vi "LEIN to Encapsulation.vi"(0 "LEIN Variation":T1, 7 "CMD":T2={"SID"=0, "ANF"=FALSE, "CMD"=enum."TASK", "DATA"=[]}, 11 "error in (no error)":errorcluster) -> (2 "Header":u16, 3 "Data":u8[](array[numeric]), 8 "Data and header":u8[](array[numeric]), 14 "Data Length":u32, 15 "error out":errorcluster)   [LabVIEW 2011]
uses:
  Defenitions/LEIN CMD Cluster.ctl
  Defenitions/LEIN CMD List.ctl
  Defenitions/LEIN Structure variations.ctl
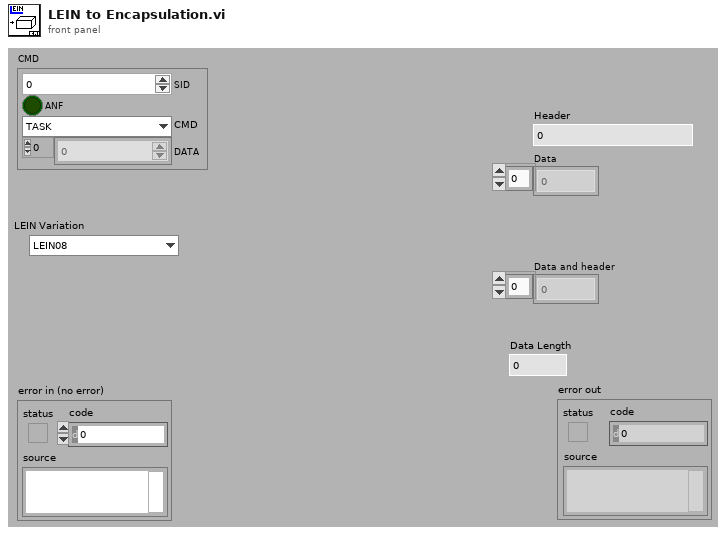
[diagram p1: front panel]
types:
  T1 = typedef "LEIN Structure variations.ctl" = enum16{"LEIN08", "LEIN31", "LEIN63"}
  T2 = typedef "LEIN CMD Cluster.ctl" = cluster{"SID":u8, "ANF":bool, "CMD":T3, "DATA":u8[]}
  T3 = typedef "LEIN CMD List.ctl" = enum8{"ACTI", "TASK", "RES0", "STAT", "RES1", "RES2", "RES3", "USER"}
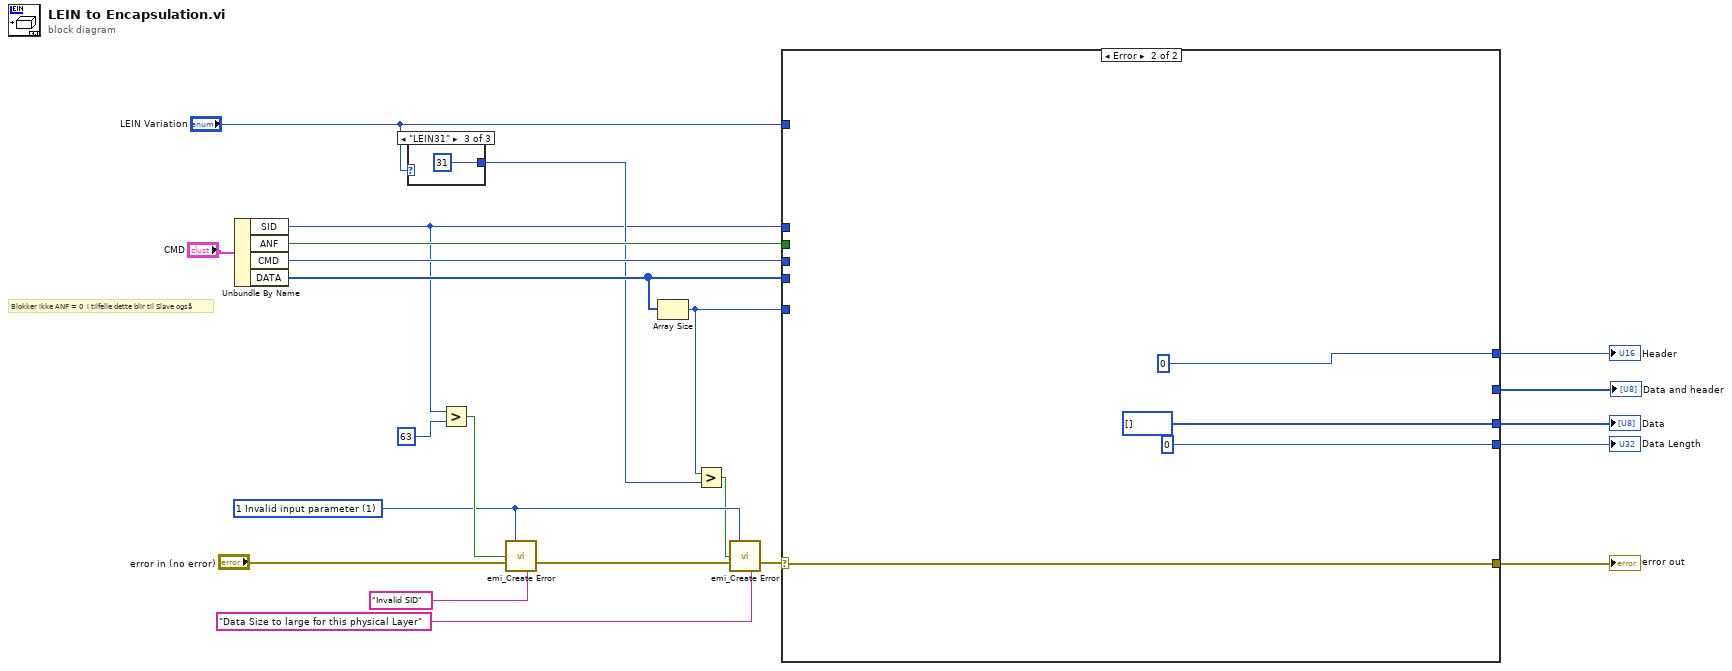
[diagram p0: block diagram]
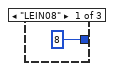
[diagram p2: hidden frame]
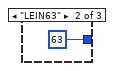
[diagram p3: hidden frame]
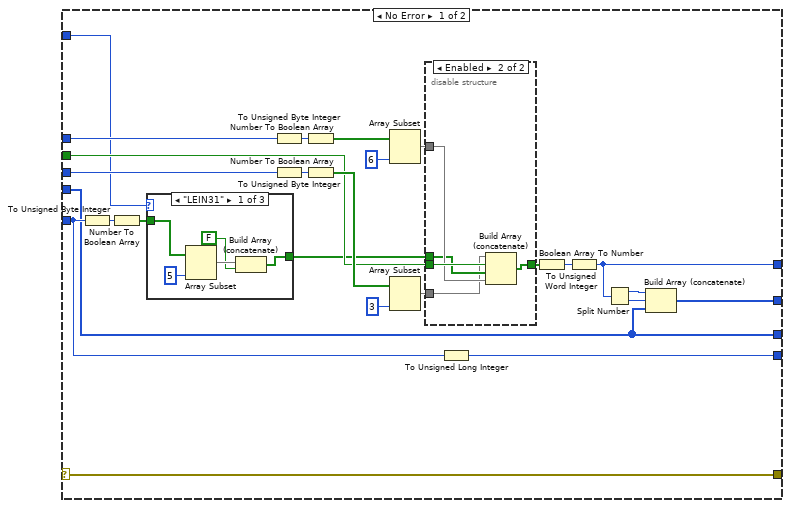
[diagram p4: hidden frame]
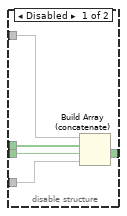
[diagram p5: hidden frame]
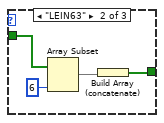
[diagram p6: hidden frame]
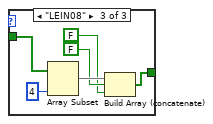
[diagram p7: hidden frame]
diagram:
  w13 = 1 items=["0 No Error"=0, "1 Invalid input parameter"=1, "6 Generic file IO "=6, "7 File not Found"=7, "35 Generic Pring Error"=35, "37 Device not Found"=37, "39 Device Unit Error"=39, "40 Could fot Open Device"=40, "42 Generic Error"=42, "52 Unknown Message"=52, "98 Bad File type"=98, "99 Bad File Version"=99, "100 Bad Data in File"=100, "1018 Unspecefied Error"=1018, "1041 Incorrect Password"=1041, "1043 Feature not in this version"=1043, "1109 Unsuported Data type"=1109, "1444 Did not close sucessfully"=1444] ("Error Code")
  # "Blokker ikke ANF = 0  i tilfelle dette blir til Slave også"
  n1 = Unbundle By Name("CMD") -> ("SID"=w1:u8, "ANF"=w20:bool, "CMD"=w16:T3, "DATA"=w6:u8[])
  n2 = case shown="\"LEIN31\"" "LEIN Variation" {
    tunnel: [8 ("y") 63 ("y") 31 ("y")] -> w4
    frame "LEIN08" {
    }
    frame "LEIN63" {
    }
    frame "LEIN31" {
    }
  }
  n3 = Greater?(x=w1, y=u8 63) -> (0:w17:bool)
  n4 = call "emi_Create Error.vi"("Error Code"=w13, "Error(T)"=w17, "error in (no error)"="error in (no error)", "Append String(\"\")"="Invalid SID" ("Append String(\"\")")) -> ("error out"=w14:errorcluster)  [unwired: 11 in]
  n5 = Array Size(array=w6) -> (size(s)=w12:i32)
  n6 = Greater?(x=w12, y=w4) -> (0:w11:bool)
  n7 = call "emi_Create Error.vi"("Error Code"=w13, "Error(T)"=w11, "error in (no error)"=w14, "Append String(\"\")"="Data Size to large for this physical Layer" ("Append String(\"\")")) -> ("error out"=w9:errorcluster)  [unwired: 11 in]
  n8 = case shown="Error" w9 {
    selector: w9 -> [w43 w79]
    tunnel: [w33 u16 0] -> w21
    tunnel: w20 -> [w39 _]
    tunnel: w16 -> [w45 _]
    tunnel: w1 -> [w44 _]
    tunnel: w12 -> [w36 _]
    tunnel: [w43 w79] -> w8
    tunnel: [w40 u32 0] -> w7
    tunnel: w6 -> [w30 _]
    tunnel: [w30 u8[] [] ("DATA")] -> w5
    tunnel: "LEIN Variation" -> [w38 _]
    tunnel: [w29 _] -> w2
    frame No Error {
      n9 = To Unsigned Byte Integer(number=w36) -> (unsigned 8bit integer=w37:u8)
      n10 = Number To Boolean Array(number=w37) -> (Boolean array=w35:bool[])
      n11 = case shown="\"LEIN31\"" w38 {
        tunnel: w35 -> [w65 w69 w75]
        tunnel: [w62 w66 w72] -> w34
        frame "LEIN31" {
          n12 = Array Subset(array=w65, length=5) -> (w63:bool[])  [unwired: 1 in]
          n13 = Build Array (concatenate)(w63, FALSE) -> (w62:bool[])
        }
        frame "LEIN63" {
          n14 = Array Subset(array=w69, length=6) -> (w67:bool[])  [unwired: 1 in]
          n15 = Build Array (concatenate)(w67) -> (w66:bool[])
        }
        frame "LEIN08" {
          n16 = Array Subset(array=w75, length=4) -> (w73:bool[])  [unwired: 1 in]
          n17 = Build Array (concatenate)(w73, FALSE, FALSE) -> (w72:bool[])
        }
      }
      n18 = To Unsigned Byte Integer(number=w44) -> (unsigned 8bit integer=w49:u8)
      n19 = To Unsigned Byte Integer(number=w45) -> (unsigned 8bit integer=w50:u8)
      n20 = Number To Boolean Array(number=w49) -> (Boolean array=w47:bool[])
      n21 = Number To Boolean Array(number=w50) -> (Boolean array=w48:bool[])
      n22 = Array Subset(array=w47, length=6) -> (w27:bool[])  [unwired: 1 in]
      n23 = Array Subset(array=w48, length=3) -> (w26:bool[])  [unwired: 1 in]
      n24 = disable-structure shown="Enabled" {
        disable-tunnel: [w55 w60] -> w42
        disable-tunnel: w39 -> [w54 w59]
        disable-tunnel: w34 -> [w53 w57]
        disable-tunnel: w27 -> [w52 w58]
        disable-tunnel: w26 -> [w51 w56]
        frame Disabled {
          n25 = Build Array (concatenate)(w52, w53, w54, w51) -> (w55:bool[])
        }
        frame Enabled {
          n26 = Build Array (concatenate)(w56, w59, w57, w58) -> (w60:bool[])
        }
      }
      n27 = To Unsigned Long Integer(number=w36) -> (unsigned 32bit integer=w40:u32)
      n28 = Boolean Array To Number(Boolean array=w42) -> (number=w41:u32)
      n29 = To Unsigned Word Integer(number=w41) -> (unsigned 16bit integer=w33:u16)
      n30 = Split Number(x=w33) -> (hi(x)=w32:u8, lo(x)=w31:u8)
      n31 = Build Array (concatenate)(w32, w31, w30) -> (w29:u8[])
    }
    frame Error {
    }
  }
  "Header" <- w21
  "Data Length" <- w7
  "error out" <- w8
  "Data" <- w5
  "Data and header" <- w2
